vi "Palindrome Checker.vi"(11 "Numeric":dbl) -> (3 "Is Palindromic Number":bool)   [LabVIEW 2025]
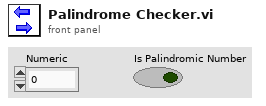
[diagram p1: front panel]
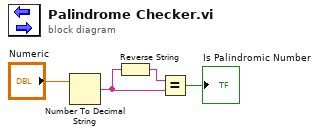
[diagram p0: block diagram]
diagram:
  n1 = Number To Decimal String(number="Numeric") -> (decimal integer string=w3:string)  [unwired: 1 in]
  n2 = Reverse String(1:w3) -> (0:w2:string)
  n3 = Equal?(x=w2, y=w3) -> (x = y?=→"Is Palindromic Number":bool)
